vi "svc_Format Value (DBL).vi"(8 "number format":i16(ring) items=["Engineering", "Exponential", "Fractional", "Automatic"], 9 "precision (1)":i16=1, 10 "width (-)":i16, 11 "dB reference":dbl=2e-05) -> (3 "format string":string)   [LabVIEW 2017]
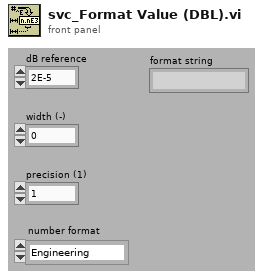
[diagram p1: front panel]
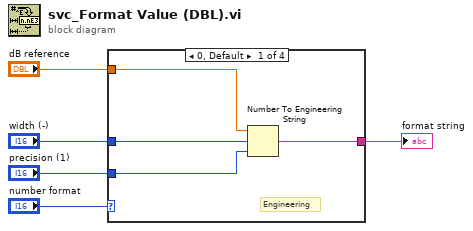
[diagram p0: block diagram]
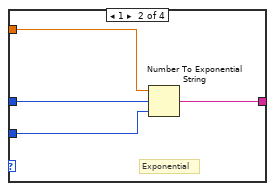
[diagram p2: hidden frame]
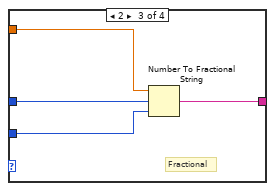
[diagram p3: hidden frame]
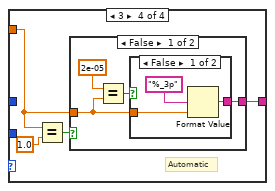
[diagram p4: hidden frame]
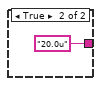
[diagram p5: hidden frame]
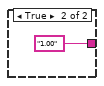
[diagram p6: hidden frame]
diagram:
  n1 = case shown="0, Default" "number format" {
    tunnel: [w7 w13 w17 w21] -> w2
    tunnel: "width (-)" -> [w8 w12 w16 _]
    tunnel: "precision (1)" -> [w9 w11 w15 _]
    tunnel: "dB reference" -> [w6 w10 w14 w20]
    frame 0, Default {
      # "Engineering"
      n2 = Number To Engineering String(2:w9, 3:w8, 4:w6) -> (0:w7:string)  [unwired: 1 in]
    }
    frame 1 {
      # "Exponential"
      n3 = Number To Exponential String(number=w10, precision (6)=w11, 3:w12) -> (E-format string=w13:string)  [unwired: 1 in]
    }
    frame 2 {
      # "Fractional"
      n4 = Number To Fractional String(number=w14, width (-)=w16, precision (6)=w15) -> (F-format string=w17:string)  [unwired: 1 in]
    }
    frame 3 {
      # "Automatic"
      n5 = Equal?(x=w20, y=1.0) -> (x = y?=w18:bool)
      n6 = case shown="False" w18 {
        tunnel: [w25 "1.00" ("format string")] -> w21
        tunnel: w20 -> [w24 _]
        frame False {
          n7 = Equal?(x=2e-05 ("y"), y=w24) -> (x = y?=w22:bool)
          n8 = case shown="False" w22 {
            tunnel: [w27 "20.0u" ("format string")] -> w25
            tunnel: w24 -> [w26 _]
            frame False {
              n9 = Format Value(format string="%_3p", value (0)=w26) -> (output string=w27:string)  [unwired: 1 in]
            }
            frame True {
            }
          }
        }
        frame True {
        }
      }
    }
  }
  "format string" <- w2
